vi "add_AccelWithCovariance.vi"(6 "AccelCovariance":T1={"Vector"={"Linear"={"x"=0.0, "y"=0.0, "z"=0.0}, "Angular"={"x"=0.0, "y"=0.0, "z"=0.0}}, "Covariance"=[0.0, 0.0, 0.0, 0.0, 0.0]}, 7 "msg in":string) -> (3 "msg out":string)   [LabVIEW 2015]
uses:
  std_msgs/subs/float64Array.vi
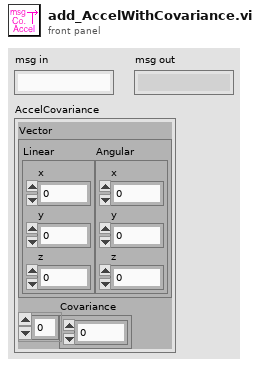
[diagram p1: front panel]
types:
  T1 = cluster{"Vector":cluster{"Linear":cluster{"x":dbl, "y":dbl, "z":dbl}, "Angular":cluster{"x":dbl, "y":dbl, "z":dbl}}, "Covariance":dbl[]}
  T2 = cluster{"Linear":cluster{"x":dbl, "y":dbl, "z":dbl}, "Angular":cluster{"x":dbl, "y":dbl, "z":dbl}}
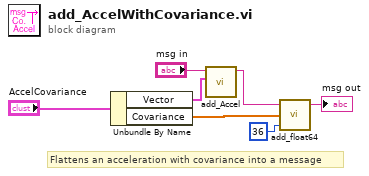
[diagram p0: block diagram]
diagram:
  # "Flattens an acceleration with covariance into a message"
  n1 = Unbundle By Name("AccelCovariance") -> ("Vector"=w2:T2, "Covariance"=w1:dbl[])
  n2 = call "add_Accel.vi"("Accel"=w2, "msg in"="msg in") -> ("msg out"=w4:string)  [unwired: 5 in]
  n3 = call-poly "add_float64.vi"("Array Length"=36, "Array"=w1, "msg in"=w4) -> ("msg out"=→"msg out":string)  [unwired: 2 in]
